vi "DraadtoevoerMachine_backup.vi"() -> ()   [LabVIEW 2013]
panel:
  out "sum":dbl
  in  "Tab Control":enum32{"Runtime operation", "Settings"}(tab)
  out "Extruded length":dbl(graph)
  out "Temperature log Next Spindle":dbl[](graph)
  out "Temperature log Current Spindle":dbl[](graph)
  in  "Emergency Button":bool
  out "SimulateWarning":string
  in  "Next spindle Type":string(combo)="Big 5[mm]"
  in  "Temperature set point [C]":dbl format="%#_3g"
  out "Next Spindel change [min]":cluster{dbl, dbl}(knob)={0.0, 7.436805212283668} scale=0.0..10.0
  in  "Current spindle Type":string(combo)="Big 5[mm]"
  in  "Temperature set point [C]":dbl format="%#_3g"
  out "Actual Temp next":dbl(slide) scale=0.0..100.0
  in  "Administrator password":string
  in  "stop":bool
  in  "Length set point [mm]":dbl=3000.0 format="%#_3g"
  out "Error Out":errorcluster
  in  "Min length alarm":dbl
  in  "Temp low Deviation":dbl
  in  "Temp high Deviation":dbl
  in  "Run Simulation":bool
  in  "DenProces 2":dbl[](array[numeric])
  in  "NumProcess 2":dbl[](array[numeric])
  in  "DenProces":dbl[](array[numeric])=[2.939e+25, 1.36e+27, 4.08e+27]
  in  "NumProcess":dbl[](array[numeric])=[0.0, 1.36e+27, 4.08e+27]
  # "Length Transfer Function"
  # "U"
  # "Omega"
  # "Heat Transfer Function"
  # "U"
  # "Temperature"
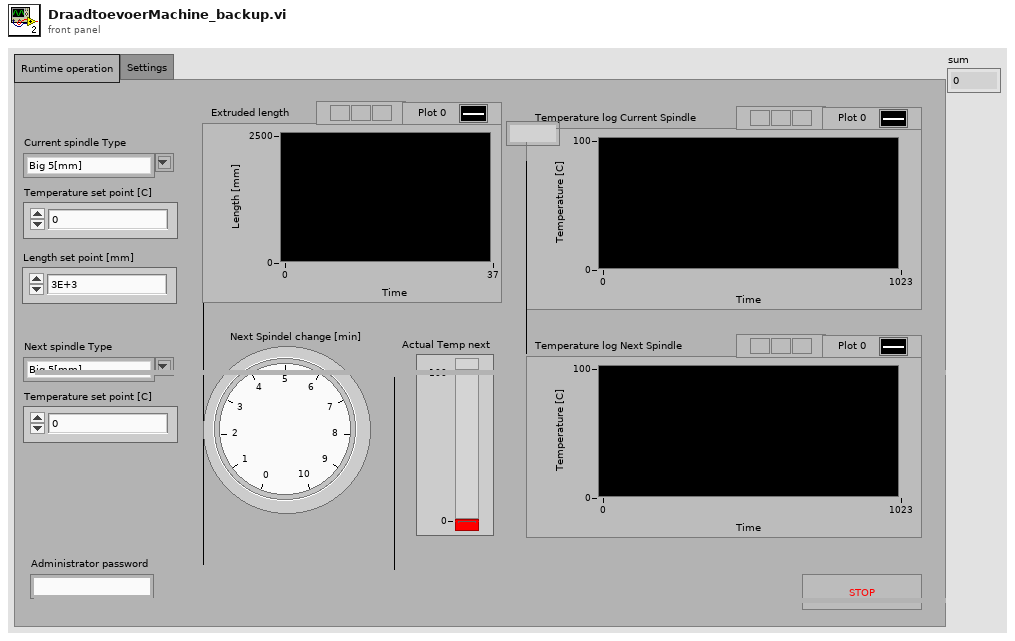
[diagram p1: front panel]
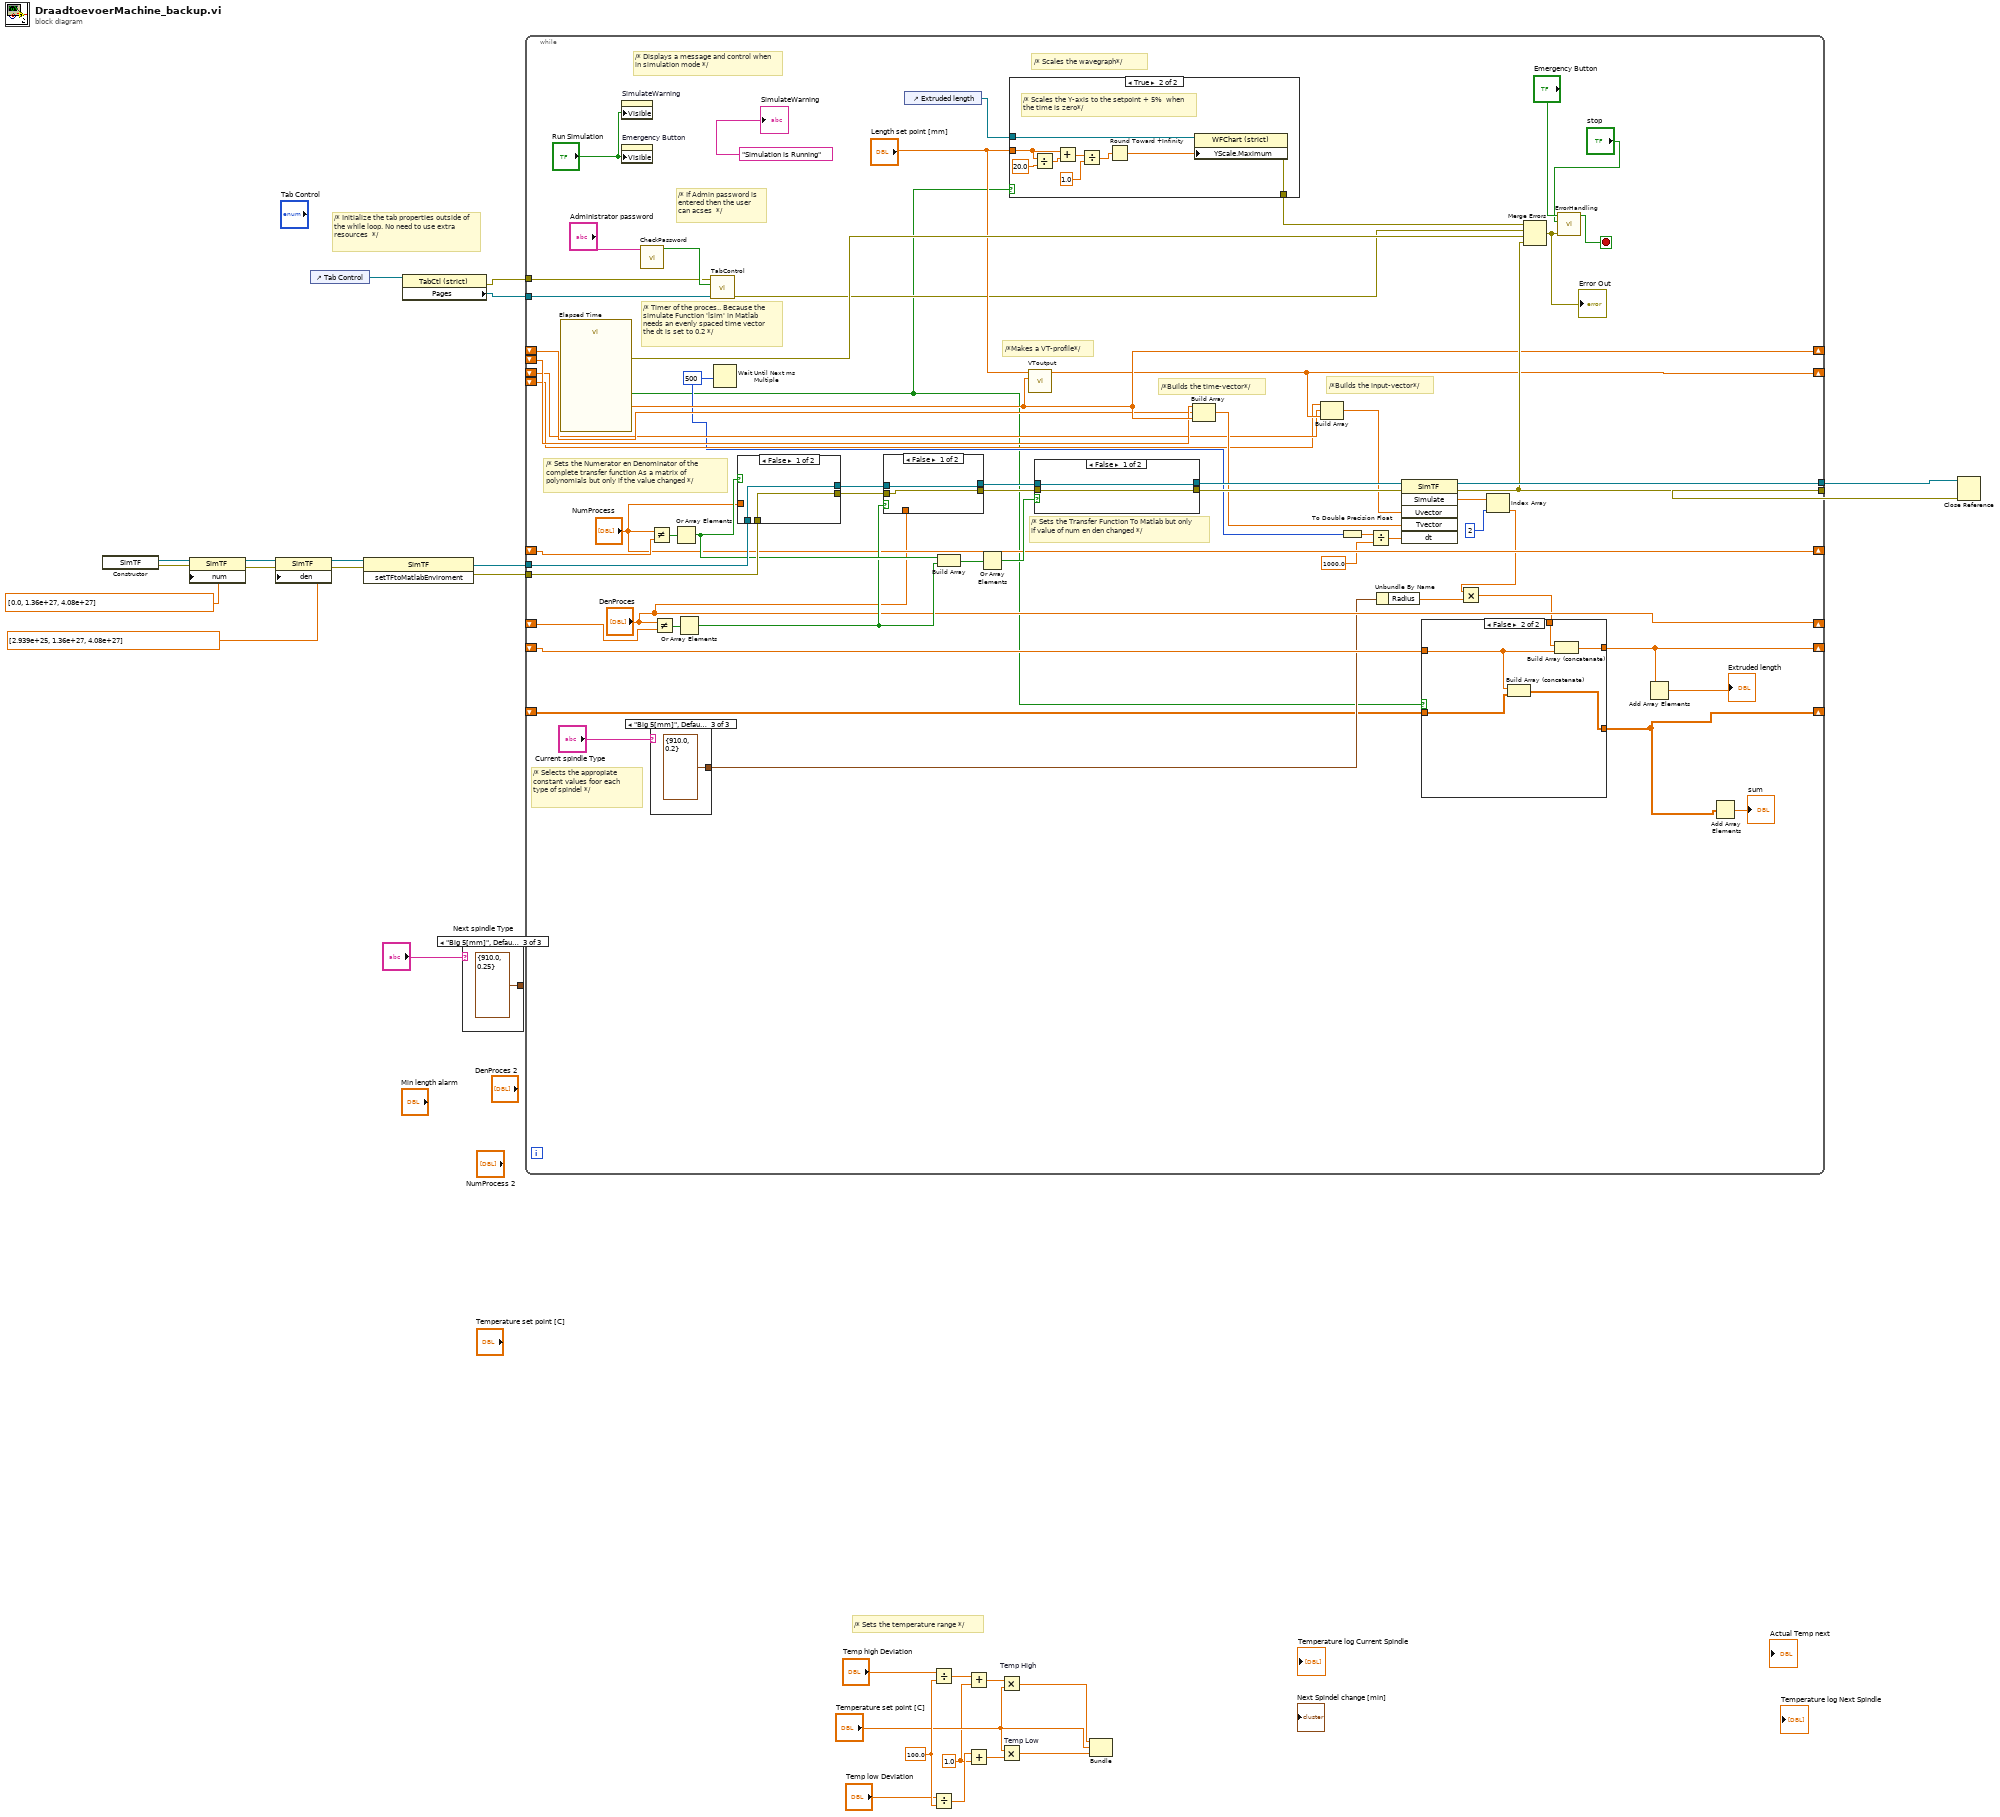
[diagram p0: block diagram]
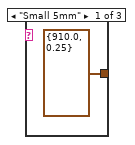
[diagram p2: hidden frame]
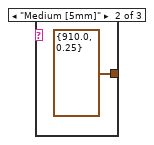
[diagram p3: hidden frame]
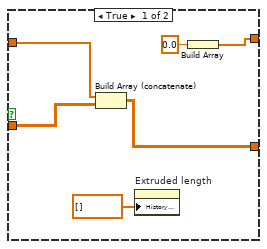
[diagram p4: hidden frame]
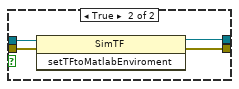
[diagram p6: hidden frame]
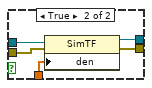
[diagram p7: hidden frame]
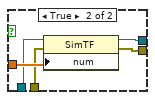
[diagram p8: hidden frame]
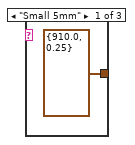
[diagram p9: hidden frame]
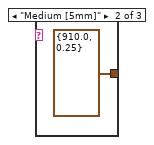
[diagram p10: hidden frame]
diagram:
  w23 = 100.0 ("y")
  w13 = 1.0 ("y")
  # "/* Sets the temperature range */"
  # "/* Initialize the tab properties outside of the while loop. No need to use extra resources  */"
  n1 = constructor class="SimTF"() -> (reference out=w8:refnum<k24>, error out=w7:errorcluster)  [unwired: 3 in, 1 out]
  n2 = property class="SimTF"(reference=w8, error in=w7, "num"=dbl[] [0.0, 1.36e+27, 4.08e+27]) -> (reference out=w10:refnum<k24>, error out=w9:errorcluster)
  n3 = property class="SimTF"(reference=w10, error in=w9, "den"=dbl[] [2.939e+25, 1.36e+27, 4.08e+27]) -> (reference out=w4:refnum<k24>, error out=w3:errorcluster)
  n4 = control-ref of="Tab Control"() -> (w27:refnum<vi>)
  n5 = invoke class="SimTF" method="setTFtoMatlabEnviroment"(reference=w4, error in=w3) -> (reference out=w2:refnum<k24>, error out=w1:errorcluster)  [unwired: 1 in, 1 out]
  n6 = property class="TabCtl (strict)"(reference=w27) -> (error out=w25:errorcluster, "Pages"=w26:refnum<vi>[])  [unwired: 1 in, 1 out]
  n7 = case shown="\"Big 5[mm]\", Default" "Next spindle Type" {
    tunnel: [cluster{"Weight":dbl, "Radius":dbl} {"Weight"=910.0, "Radius"=0.25} cluster{"Weight":dbl, "Radius":dbl} {"Weight"=910.0, "Radius"=0.25} cluster{"Weight":dbl, "Radius":dbl} {"Weight"=910.0, "Radius"=0.25}] -> _
    frame "Small 5mm" {
    }
    frame "Medium [5mm]" {
    }
    frame "Big 5[mm]", Default {
    }
  }
  n8 = while {
    tunnel: w26 -> [w82]
    tunnel: w1 -> [w77]
    tunnel: w2 -> [w76]
    tunnel: w25 -> [w81]
    tunnel: [w61] -> w24
    shift-right: ["NumProcess"] -> _
    shift-left: _ -> [w79]
    shift-right: ["DenProces"] -> _
    shift-left: _ -> [w75]
    tunnel: [w62] -> w11
    shift-right: [w50] -> _
    shift-left: _ -> [w49]
    shift-right: [w53] -> _
    shift-left: _ -> [w51]
    shift-left: _ -> [w52]
    shift-left: _ -> [w48]
    shift-right: [w34] -> _
    shift-left: _ -> [w41]
    shift-right: [w32] -> _
    shift-left: _ -> [w33]
    stop <- w83 stop-if-true
    w43 = u32 500 ("millisecond multiple")
    # "/*Builds the input-vector*/"
    # "/*Builds the time-vector*/"
    # "/*Makes a VT-profile*/"
    # "/* Scales the wavegraph*/"
    # "/* Timer of the proces.. Because the simulate Function 'lsim' in Matlab needs an evenly spaced time vector the dt is set to 0.2 */"
    # "/* Sets the Transfer Function To Matlab but only if value of num en den changed */"
    # "/* If Admin password is entered then the user can acses  */"
    # "/* Sets the Numerator en Denominator of the complete transfer function As a matrix of polynomials but only if the value changed */"
    # "/* Displays a message and control when in simulation mode */"
    # "/* Selects the appropiate constant values foor each type of spindel */"
    n9 = call "Elapsed Time"() -> ("Elapsed Time (s)"=w53:dbl, "Time has Elapsed"=w36:bool, "error out"=w80:errorcluster)  [unwired: 12 in, 5 out]
    n10 = property on="SimulateWarning" class="Str"("Visible"="Run Simulation") -> ()  [unwired: 2 in, 2 out]
    n11 = property on="Emergency Button" class="Bool (strict)"("Visible"="Run Simulation") -> ()  [unwired: 2 in, 2 out]
    n12 = call "CheckPassword.vi"("Administrator password"="Administrator password") -> ("Boolean"=w88:bool)  [unwired: 10 in]
    n13 = Not Equal?(x="NumProcess", y=w79) -> (x != y?=w78:bool[])
    n14 = case shown="\"Big 5[mm]\", Default" "Current spindle Type" {
      tunnel: [cluster{"Weight":dbl, "Radius":dbl} {"Weight"=910.0, "Radius"=0.25} cluster{"Weight":dbl, "Radius":dbl} {"Weight"=910.0, "Radius"=0.25} cluster{"Weight":dbl, "Radius":dbl} {"Weight"=910.0, "Radius"=0.2}] -> w40
      frame "Small 5mm" {
      }
      frame "Medium [5mm]" {
      }
      frame "Big 5[mm]", Default {
      }
    }
    n15 = Not Equal?(x="DenProces", y=w75) -> (x != y?=w74:bool[])
    n16 = Or Array Elements(Boolean array=w78) -> (logical OR=w68:bool)
    n17 = Or Array Elements(Boolean array=w74) -> (logical OR=w67:bool)
    n18 = call "TabControl.vi"("Pages"=w82, "Boolean"=w88, "error in (no error)"=w81) -> ("error out"=w57:errorcluster)  [unwired: 8 in]
    n19 = Wait Until Next ms Multiple(millisecond multiple=w43) -> ()  [unwired: 1 out]
    n20 = case shown="False" w68 {
      tunnel: w77 -> [w125 w127]
      tunnel: w76 -> [w126 w128]
      tunnel: [w126 w131] -> w73
      tunnel: [w125 w130] -> w72
      tunnel: "NumProcess" -> [_ w129]
      frame False {
      }
      frame True {
        n21 = property class="SimTF"(reference=w128, error in=w127, "num"=w129) -> (reference out=w131:refnum<k24>, error out=w130:errorcluster)
      }
    }
    n22 = case shown="False" w67 {
      tunnel: w73 -> [w119 w124]
      tunnel: w72 -> [w118 w123]
      tunnel: "DenProces" -> [_ w122]
      tunnel: [w119 w121] -> w71
      tunnel: [w118 w120] -> w70
      frame False {
      }
      frame True {
        n23 = property class="SimTF"(reference=w124, error in=w123, "den"=w122) -> (reference out=w121:refnum<k24>, error out=w120:errorcluster)
      }
    }
    n24 = control-ref of="Extruded length"() -> (w59:refnum<vi>)
    n25 = Build Array(w68, w67) -> (w69:bool[])
    n26 = Or Array Elements(Boolean array=w69) -> (logical OR=w66:bool)
    n27 = case shown="True" w36 {
      tunnel: [_ w111] -> w56
      tunnel: "Length set point [mm]" -> [_ w110]
      tunnel: w59 -> [_ w104]
      frame False {
      }
      frame True {
        # "/* Scales the Y-axis to the setpoint + 5%  when the time is zero*/"
        n28 = Divide(x=w110, y=20.0) -> (x/y=w108:dbl)
        n29 = Add(x=w110, y=w108) -> (x+y=w107:dbl)
        n30 = Divide(x=w107, y=1.0) -> (x/y=w106:dbl)
        n31 = Round Toward +Infinity(x=w106) -> (ceil(x): smallest int >= x=w103:dbl)
        n32 = property on="Property Node" class="WFChart (strict)"(reference=w104, "YScale.Maximum"=w103) -> (error out=w111:errorcluster)  [unwired: 1 in, 1 out]
      }
    }
    n33 = call "VToutput.vi"("Elapsed Time (s)"=w53, "Length set point [mm]"="Length set point [mm]") -> ("V"=w50:dbl)  [unwired: 9 in]
    n34 = case shown="False" w66 {
      tunnel: w71 -> [w113 w117]
      tunnel: w70 -> [w112 w116]
      tunnel: [w113 w115] -> w65
      tunnel: [w112 w114] -> w64
      frame False {
      }
      frame True {
        n35 = invoke class="SimTF" method="setTFtoMatlabEnviroment"(reference=w117, error in=w116) -> (reference out=w115:refnum<k24>, error out=w114:errorcluster)  [unwired: 1 in, 1 out]
      }
    }
    n36 = Build Array(w52, w51, w53) -> (w63:dbl[])
    n37 = Build Array(w48, w49, w50) -> (w60:dbl[])
    n38 = To Double Precision Float(number=w43) -> (double precision float=w44:dbl)
    n39 = Divide(x=w44, y=1000.0) -> (x/y=w45:dbl)
    n40 = Unbundle By Name(w40) -> ("Radius"=w39:dbl)
    n41 = invoke class="SimTF" method="Simulate"(reference=w65, error in=w64, "Uvector"=w60, "Tvector"=w63, "dt"=w45) -> (reference out=w62:refnum<k24>, error out=w61:errorcluster, "Simulate"=w47:dbl[])  [unwired: 1 in, 3 out]
    n42 = Index Array(array=w47, index=2) -> (element=w38:dbl)
    n43 = Multiply(x=w38, y=w39) -> (x*y=w37:dbl)
    n44 = case shown="False" w36 {
      tunnel: [w96 w102] -> w34
      tunnel: w41 -> [w94 w100]
      tunnel: w37 -> [_ w101]
      tunnel: [w93 w98] -> w32
      tunnel: w33 -> [w92 w99]
      frame True {
        n45 = Build Array (concatenate)(w94, w92) -> (w93:dbl[][])
        n46 = property on="Extruded length" class="WFChart (strict)"("History Data"=dbl[] []) -> ()  [unwired: 2 in, 2 out]
        n47 = Build Array(0.0 ("element")) -> (w96:dbl[])
      }
      frame False {
        n48 = Build Array (concatenate)(w100, w99) -> (w98:dbl[][])
        n49 = Build Array (concatenate)(w101, w100) -> (w102:dbl[])
      }
    }
    n50 = Merge Errors(w56, w57, w80, w61) -> (w84:errorcluster)
    "Error Out" <- w84
    n51 = call "ErrorHandling.vi"("error in (no error)"=w84, "stop"="stop", "Emergency Button"="Emergency Button") -> ("Boolean"=w83:bool)  [unwired: 8 in]
    n52 = Add Array Elements(numeric array=w34) -> (sum=→"Extruded length":dbl)
    n53 = Add Array Elements(numeric array=w32) -> (sum=→"sum":dbl)
    "SimulateWarning" <- "Simulation is Running" ("SimulateWarning")
  }
  n54 = Divide(x="Temp high Deviation", y=w23) -> (x/y=w19:dbl)
  n55 = Divide(x="Temp low Deviation", y=w23) -> (x/y=w21:dbl)
  n56 = Add(x=w19, y=w13) -> (x+y=w14:dbl)
  n57 = Add(x=w21, y=w13) -> (x+y=w15:dbl)
  n58 = Multiply "Temp High"(x=w14, y="Temperature set point [C]") -> (x*y=w16:dbl)
  n59 = Multiply "Temp Low"(x="Temperature set point [C]", y=w15) -> (x*y=w18:dbl)
  n60 = Bundle(w16, "Temperature set point [C]"="Temperature set point [C]", w18) -> ()  [unwired: 1 in, 1 out]
  n61 = Close Reference(reference=w11, error in (no error)=w24) -> ()  [unwired: 1 out]
